vi "Byte Buffer.Mapping.Get Sizes.vi"(11 "mappings":T1[](array[typedef])) -> (0 "largest double count":i32, 1 "largest mapping size":i32, 2 "total sequential size":i32, 3 "required buffer size":i32)   [LabVIEW 2016]
uses:
  Byte Buffer.Mapping.ctl
  Typedefs/Typedefs.Data Types.ctl
  SubVIs/Sizeof.Scalar.vi
  VeriStand Data.lvlib
  Byte Buffer.lvclass
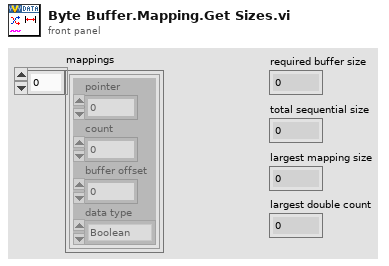
[diagram p1: front panel]
types:
  T1 = typedef "VeriStand Data.lvlib/Byte Buffer.lvclass/Byte Buffer.Mapping.ctl" = cluster{"pointer":u64, "count":i32, "buffer offset":i32, "data type":T2}
  T2 = typedef "VeriStand Data.lvlib/Typedefs.Data Types.ctl" = enum16{"Boolean", "Single", "Double", "I8", "I16", "I32", "I64", "U8", "U16", "U32", "U64"}
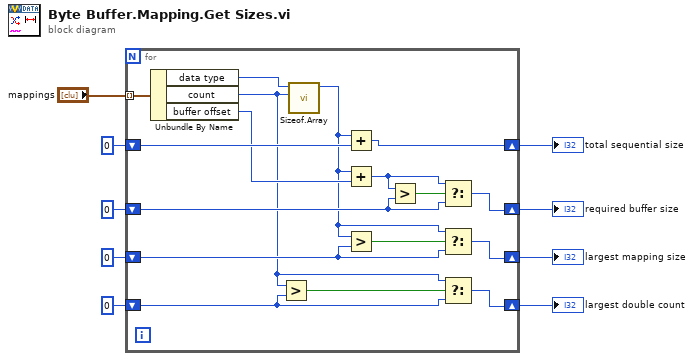
[diagram p0: block diagram]
diagram:
  n1 = for {
    tunnel: "mappings" -> [w26] mode=indexing
    shift-right: [w24] -> w8
    shift-left: 0 -> [w23]
    shift-right: [w19] -> w5
    shift-left: 0 -> [w20]
    shift-right: [w16] -> w3
    shift-left: 0 -> [w15]
    shift-right: [w13] -> w1
    shift-left: 0 -> [w12]
    n2 = Unbundle By Name(w26) -> ("data type"=w25:T2, "count"=w10:i32, "buffer offset"=w22:i32)
    n3 = Greater?(x=w10, y=w12) -> (0:w11:bool)
    n4 = call "Sizeof.Array.vi"("count"=w10, "data type"=w25) -> ("size"=w17:i32)  [unwired: 9 in]
    n5 = Add(x=w17, y=w23) -> (x+y=w24:i32)
    n6 = Add(x=w17, y=w22) -> (x+y=w14:i32)
    n7 = Greater?(x=w17, y=w15) -> (0:w18:bool)
    n8 = Greater?(x=w14, y=w20) -> (0:w21:bool)
    n9 = Select(t=w14, s=w21, f=w20) -> (s? t:f=w19:i32)
    n10 = Select(t=w17, s=w18, f=w15) -> (s? t:f=w16:i32)
    n11 = Select(t=w10, s=w11, f=w12) -> (s? t:f=w13:i32)
  }
  "total sequential size" <- w8
  "largest mapping size" <- w3
  "required buffer size" <- w5
  "largest double count" <- w1
